vi "specu1a 1.0.0 Write Parameters.vi"(4 "Parameters":T1={"Integration time"=10000, "Gain"=enum."Low", "TriggerEdge"=enum."Rising", "Trigger Mode"=enum."Internal", "Reserved"=0}, 5 "Device Handle":i32) -> (1 "Parameters out":T1={"Integration time"=10000, "Gain"=enum."Low", "TriggerEdge"=enum."Rising", "Trigger Mode"=enum."Internal", "Reserved"=0}, 2 "Device Handle out":i32)   [LabVIEW 2019]
uses:
  Controls/specu1a 1.0.0 Parameters.ctl
  Controls/specu1a 1.0.0 Trigger Edge.ctl
  Controls/specu1a 1.0.0 Trigger Mode.ctl
  specu1a.dll
panel:
  in  "error IO 2":errorcluster
  out "error IO":errorcluster
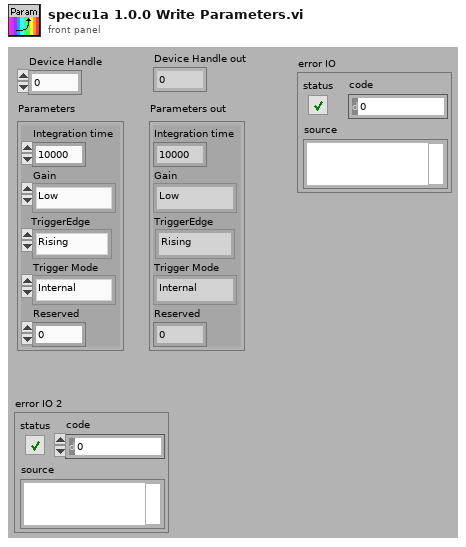
[diagram p1: front panel]
types:
  T1 = typedef "specu1a 1.0.0 Parameters.ctl" = cluster{"Integration time":u32, "Gain":enum16{"Low", "High", "No Function"}, "TriggerEdge":T2, "Trigger Mode":T3, "Reserved":u8}
  T2 = typedef "specu1a 1.0.0 Trigger Edge.ctl" = enum16{"Rising", "Falling", "No Function"}
  T3 = typedef "specu1a 1.0.0 Trigger Mode.ctl" = enum16{"Internal", "Asynchronous", "Synchronous"}
  T4 = cluster{"Integration time":u32, "Gain":u8, "Trigger edge":u8, "Trigger mode":u8, "Reserved":u8}
  T5 = typedef "specu1a 1.0.0 Error codes.ctl" = enum16{"INVALID_HANDLE_VALUE", "USBDEV_SUCCESS", "USBDEV_INVALID_HANDLE", "USBDEV_UNSUCCESS", "USBDEV_INVALID_VALUE", "USBDEV_CHECK_NORMAL", "USBDEV_CHECK_INVALID", "USBDEV_CHECK_REMOVE", "USBDEV_CHECK_OTHER", "USBDEV_RESET_ERROR", "USBDEV_BULKSIZE_ERROR", "USBDEV_BULK_READ_ERROR", "USBDEV_BULK_NOT_UPDATED", "USBDEV_TIME_OVER_ERROR", "USBDEV_TIME_UNDER_ERROR", "USBDEV_TIME_SET_ERROR", "USBDEV_SET_GAIN_ERROR", "USBDEV_GET_TEMP_ERROR", "USBDEV_SET_TRIGGER_ERROR", "USBDEV_RW_EEP_ADDR_ERROR", "USBDEV_RW_EEP_SIZE_ERROR", "USBDEV_RW_EEP_OVER_ERROR", "USBDEV_RW_EEP_ERROR", "UNITID_PRODUCTID_CONFLICT", "UNKNOWN_ERROR"}
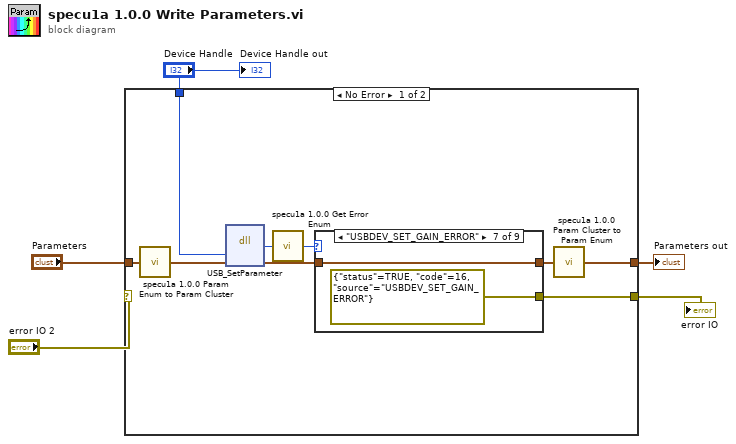
[diagram p0: block diagram]
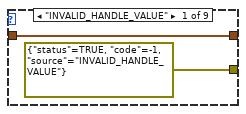
[diagram p2: hidden frame]
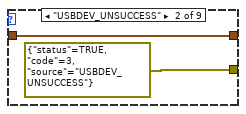
[diagram p3: hidden frame]
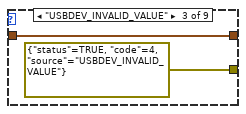
[diagram p4: hidden frame]
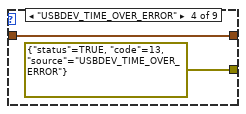
[diagram p5: hidden frame]
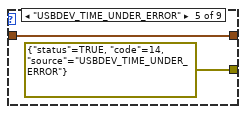
[diagram p6: hidden frame]
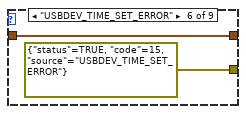
[diagram p7: hidden frame]
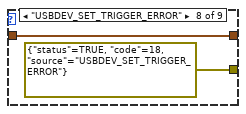
[diagram p8: hidden frame]
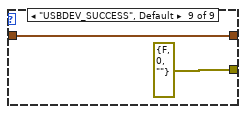
[diagram p9: hidden frame]
diagram:
  n1 = case shown="No Error" "error IO 2" {
    selector: "error IO 2" -> [_ w34]
    tunnel: [w13 w34] -> w2
    tunnel: "Device Handle" -> [w12 _]
    tunnel: "Parameters" -> [w10 w33]
    tunnel: [w6 w33] -> w3
    frame No Error {
      n2 = call "specu1a 1.0.0 Param Enum to Param Cluster.vi"("Parameters"=w10) -> ("Cluster in"=w9:T4)
      n3 = dll-call lib="C:/Users/martzlab/Desktop/SIO 179/Nitrate/64/EvaluationSoftware/minispec labview/Hamamatsu Spectrometer Dll/specu1a.dll" fn="USB_SetParameter" label="1.0.0 SetParameter"("Device Handle"=w12, "Cluster in"=w9) -> (w11:u16, "Cluster in"=w8:T4)  [unwired: 4 in, 2 out]
      n4 = call "specu1a 1.0.0 Get Error Enum.vi"("Error Code in"=w11) -> ("Specu1a 1.0.0 Error code out"=w14:T5)  [unwired: 4 in]
      n5 = case shown="\"USBDEV_SET_GAIN_ERROR\"" w14 {
        tunnel: [errorcluster {"status"=TRUE, "code"=-1, "source"="INVALID_HANDLE_VALUE"} ("error out") errorcluster {"status"=TRUE, "code"=3, "source"="USBDEV_UNSUCCESS"} ("error out") errorcluster {"status"=TRUE, "code"=4, "source"="USBDEV_INVALID_VALUE"} ("error out") errorcluster {"status"=TRUE, "code"=13, "source"="USBDEV_TIME_OVER_ERROR"} ("error out") errorcluster {"status"=TRUE, "code"=14, "source"="USBDEV_TIME_UNDER_ERROR"} ("error out") errorcluster {"status"=TRUE, "code"=15, "source"="USBDEV_TIME_SET_ERROR"} ("error out") errorcluster {"status"=TRUE, "code"=16, "source"="USBDEV_SET_GAIN_ERROR"} ("error out") errorcluster {"status"=TRUE, "code"=18, "source"="USBDEV_SET_TRIGGER_ERROR"} ("error out") errorcluster {"status"=FALSE, "code"=0, "source"=""} ("error out")] -> w13
        tunnel: [w15 w17 w19 w21 w23 w25 w27 w29 w31] -> w7
        tunnel: w8 -> [w15 w17 w19 w21 w23 w25 w27 w29 w31]
        frame "INVALID_HANDLE_VALUE" {
        }
        frame "USBDEV_UNSUCCESS" {
        }
        frame "USBDEV_INVALID_VALUE" {
        }
        frame "USBDEV_TIME_OVER_ERROR" {
        }
        frame "USBDEV_TIME_UNDER_ERROR" {
        }
        frame "USBDEV_TIME_SET_ERROR" {
        }
        frame "USBDEV_SET_GAIN_ERROR" {
        }
        frame "USBDEV_SET_TRIGGER_ERROR" {
        }
        frame "USBDEV_SUCCESS", Default {
        }
      }
      n6 = call "specu1a 1.0.0 Param Cluster to Param Enum.vi"("Cluster in"=w7) -> ("Parameters"=w6:T1)
    }
    frame Error {
    }
  }
  "Parameters out" <- w3
  "error IO" <- w2
  "Device Handle out" <- "Device Handle"
